vi "PCIe Signal Routing.vi"(6 "trigger master index":i32, 8 "error in":errorcluster, 9 "sync pulse rtsi line":string="RTSI1", 10 "start trigger rtsi line":string="RTSI0", 11 "fpga interfaces in":refnum<k20>[](array[refnum])) -> (0 "error out":errorcluster, 3 "fpga interfaces out":refnum<k20>[](array[refnum]))   [LabVIEW 2018, in "GettingStarted_5775_Host.lvlib"]
uses:
  GettingStarted_5775_Host.lvlib
  <instrlib>/FlexRIO/API/Host/v1/NI FlexRIO/API/Get Property Reference - Fpga Small.vi
  <resource>/objmgr/niflexrioapi.rc
  <instrlib>/FlexRIO/API/Host/v1/NI FlexRIO API v1.lvlib
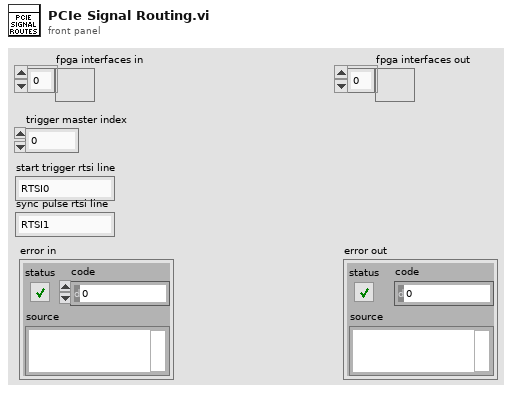
[diagram p1: front panel]
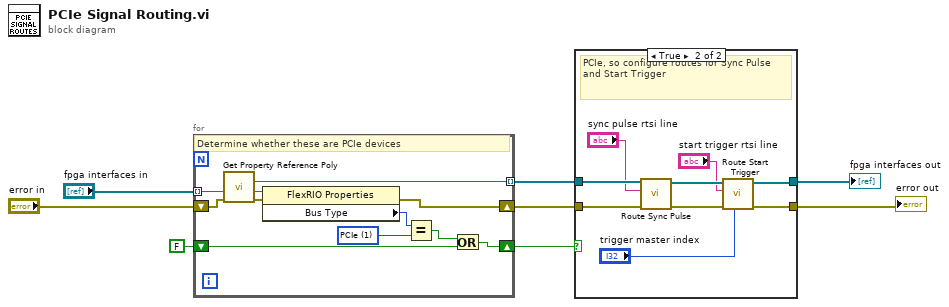
[diagram p0: block diagram]
diagram:
  n1 = for {
    tunnel: [w15] -> w8 mode=indexing
    shift-right: [w13] -> w7
    shift-left: "error in" -> [w14]
    tunnel: "fpga interfaces in" -> [w12] mode=indexing
    shift-right: [w11] -> w1
    shift-left: FALSE -> [w10]
    w17 = 1 items=["PXIe", "PCIe"] ("Description:Bus Type")
    # "Determine whether these are PCIe devices"
    n2 = call-poly <instrlib>:"Get Property Reference Poly.vi"("error in (no error)"=w14, "fpga interface in"=w12) -> ("error out"=w18:errorcluster, "property reference"=w19:refnum<k20>, "fpga interface out"=w15:refnum<k20>)  [unwired: 4 in]
    n3 = property class="FlexRIO Properties"(reference=w19, error in=w18) -> (error out=w13:errorcluster, "Bus Type"=w16:i32)  [unwired: 1 out]
    n4 = Equal?(x=w16, y=w17) -> (x = y?=w9:bool)
    n5 = Or(x=w9, y=w10) -> (x .or. y?=w11:bool)
  }
  n6 = case shown="True" w1 {
    tunnel: [w20 w25] -> w5
    tunnel: [w21 w26] -> w6
    tunnel: w8 -> [w21 w29]
    tunnel: w7 -> [w20 w30]
    frame False {
      # "Not PCIe, manual routing is not necessary"
    }
    frame True {
      # "PCIe, so configure routes for Sync Pulse and Start Trigger"
      n7 = call "Route Sync Pulse.vi"("error in"=w30, "sync pulse rtsi line"="sync pulse rtsi line", "fpga interfaces in"=w29) -> ("error out"=w28:errorcluster, "fpga interfaces out"=w27:refnum<k20>[])  [unwired: 7 in]
      n8 = call "Route Start Trigger.vi"("trigger master index"="trigger master index", "error in"=w28, "start trigger rtsi line"="start trigger rtsi line", "fpga interfaces in"=w27) -> ("error out"=w25:errorcluster, "fpga interfaces out"=w26:refnum<k20>[])  [unwired: 6 in]
    }
  }
  "fpga interfaces out" <- w6
  "error out" <- w5
